vi "GenerateAttachablePosition_Queen.vi"(1 "Black/White Turn (T/F)":bool, 2 "Board":i32[][](array[numeric])=[[-3, -5, -4, -1, -2, -4, -5, -3], [-6, -6, -6, -6, -6, -6, -6, -6], [0, 0, 0, 0, 0, 0, 0, 0], [0, 0, 0, 0, 0, 0, 0, 0], [0, 0, 0, 0, 0, 0, 0, 0], [0, 0, 0, 0, 0, 0, 0, 0], [6, 6, 6, 6, 6, 6, 6, 6], [3, 5, 4, 1, 2, 4, 5, 3]], 3 "pieceIndex":i32) -> (0 "AttachablePosition":bool[][](array[boolean]))   [LabVIEW 2014]
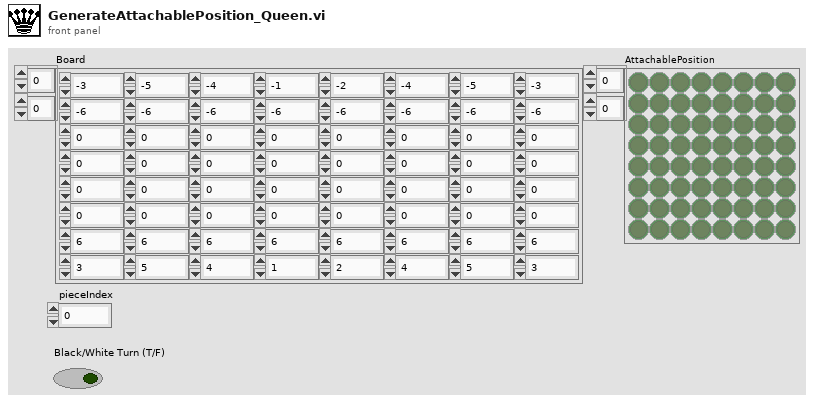
[diagram p1: front panel]
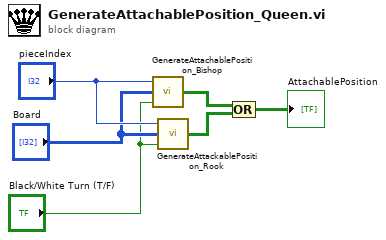
[diagram p0: block diagram]
diagram:
  n1 = call "GenerateAttachablePosition_Bishop.vi"("Black/White Turn (T/F)"="Black/White Turn (T/F)", "Board"="Board", "pieceIndex"="pieceIndex") -> ("AttachablePosition"=w5:bool[][])
  n2 = call "GenerateAttackablePosition_Rook.vi"("Black/White Turn (T/F)"="Black/White Turn (T/F)", "Board"="Board", "pieceIndex"="pieceIndex") -> ("AttachablePosition"=w1:bool[][])
  n3 = Compound Arithmetic op=OR(w5, w1) -> (→"AttachablePosition":bool[][])
